vi "Copy Class Item.vi"(8 "error in (no error)":errorcluster, 9 "New Name":string, 10 "Full path in":path, 11 "LVClassLibrary in":refnum<vi>) -> (0 "error out":errorcluster, 2 "New Class Path out":path, 3 "LVClassLibrary out":refnum<vi>)   [LabVIEW 2020, in "gRPC Scripting Tools.lvlib"]
uses:
  gRPC Scripting Tools.lvlib
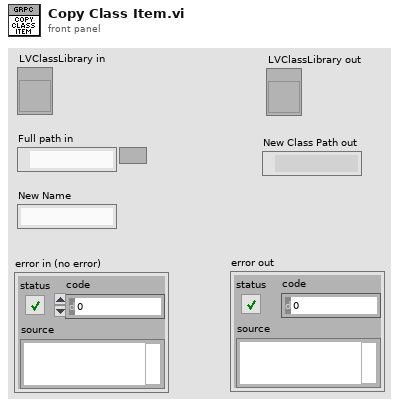
[diagram p1: front panel]
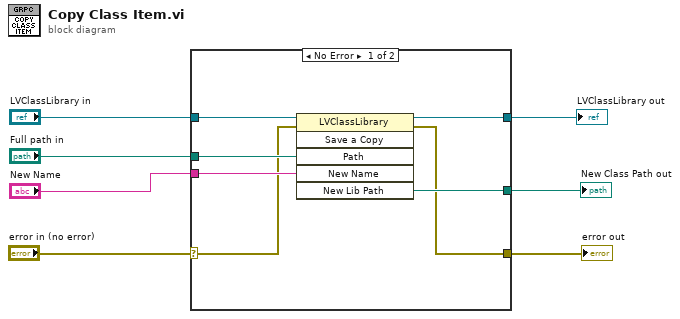
[diagram p0: block diagram]
diagram:
  n1 = case shown="No Error" "error in (no error)" {
    selector: "error in (no error)" -> [w10 w16]
    tunnel: [w14 _] -> w7
    tunnel: "New Name" -> [w13 _]
    tunnel: "Full path in" -> [w12 _]
    tunnel: "LVClassLibrary in" -> [w11 w15]
    tunnel: [w9 w16] -> w2
    tunnel: [w8 w15] -> w1
    frame No Error {
      n2 = invoke class="LVClassLibrary" method="Save a Copy"(reference=w11, error in=w10, "Path"=w12, "New Name"=w13) -> (reference out=w8:refnum<vi>, error out=w9:errorcluster, "New Lib Path"=w14:path)  [unwired: 2 in, 3 out]
    }
    frame Error {
    }
  }
  "New Class Path out" <- w7
  "error out" <- w2
  "LVClassLibrary out" <- w1
